vi "Decorate.vi"(7 "Actor":refnum<class "Actor.lvclass">) -> (5 "Decorated Actor":refnum<class "Actor.lvclass">)   [LabVIEW 2025, in "_Template.lvlib" / "Templates.lvlib" / "TEMPLATE Actor.lvlib"]
uses:
  TEMPLATE Actor.lvlib
  jettl/jettl/Actor/Actor.lvclass
  TEMPLATE Actor/TEMPLATE Actor.lvclass
  C:/git/jettl/src/jettl/jettl/Actor/Actor.lvclass
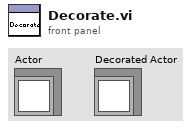
[diagram p1: front panel]
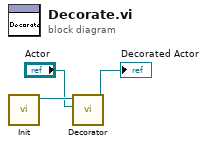
[diagram p0: block diagram]
diagram:
  n1 = call "Init.vi"() -> ("TEMPLATE Actor out"=w2:refnum<class "TEMPLATE Actor.lvclass">)  [unwired: 11 in]
  n2 = call-dynamic "Decorator.vi"("Actor"="Actor", "TEMPLATE Actor in"=w2) -> ("TEMPLATE Actor out"=→"Decorated Actor":refnum<class "TEMPLATE Actor.lvclass">)  [unwired: 9 in]
